vi "openFrontPanel.vi"(6 "Center? (True)":bool=TRUE, 8 "error in (no error)":errorcluster, 11 "VI Reference In (Top Level)":refnum<vi>) -> (0 "error out":errorcluster, 3 "VI Reference Out":refnum<vi>)   [LabVIEW 2017, in "shared.lvlib"]
uses:
  shared.lvlib
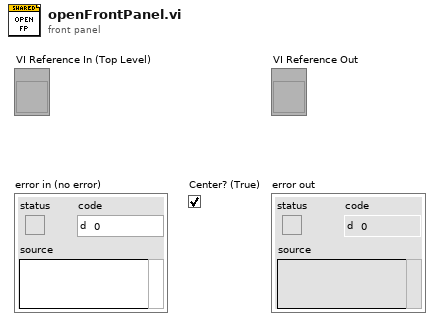
[diagram p1: front panel]
types:
  T1 = enum32{"Invalid", "Standard", "Closed", "Hidden", "Minimized", "Maximized"}
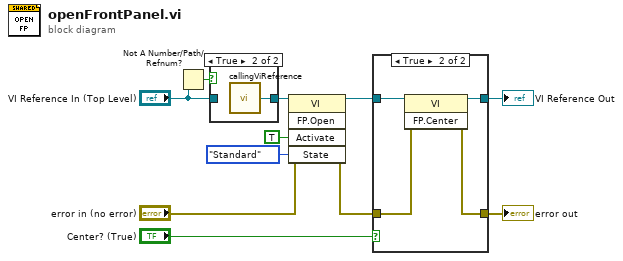
[diagram p0: block diagram]
diagram:
  n1 = Not A Number/Path/Refnum?(number/path/refnum="VI Reference In (Top Level)") -> (NaN/Path/Refnum?=w4:bool)
  n2 = case shown="True" w4 {
    tunnel: "VI Reference In (Top Level)" -> [w12 _]
    tunnel: [w12 w13] -> w2
    frame False {
    }
    frame True {
      n3 = call "callingViReference.vi"() -> ("Caller's VI Reference"=w13:refnum<vi>)  [unwired: 1 in]
    }
  }
  n4 = invoke class="VI" method="FP.Open"(reference=w2, error in="error in (no error)", "Activate"=TRUE ("Activate?"), "State"=T1."Standard") -> (reference out=w11:refnum<vi>, error out=w8:errorcluster)  [unwired: 1 in, 3 out]
  n5 = case shown="True" "Center? (True)" {
    tunnel: w11 -> [w15 w19]
    tunnel: w8 -> [w14 w18]
    tunnel: [w15 w17] -> w7
    tunnel: [w14 w16] -> w6
    frame False {
    }
    frame True {
      n6 = invoke class="VI" method="FP.Center"(reference=w19, error in=w18) -> (reference out=w17:refnum<vi>, error out=w16:errorcluster)  [unwired: 1 in, 1 out]
    }
  }
  "VI Reference Out" <- w7
  "error out" <- w6
